vi "Is VI Server Required.vi"(8 "error in (no error)":errorcluster, 11 "Timing Action in":refnum<class "Timing Action.lvclass">) -> (0 "error out":errorcluster, 2 "VI Server Required?":bool, 3 "Timing Action out":refnum<class "Timing Action.lvclass">)   [LabVIEW 2020, in "MacroAssert.lvlib" / "Timing Action.lvclass"]
doc: "Outputs whether VI Server is required to perform the given step."
uses:
  Timing Action.lvclass
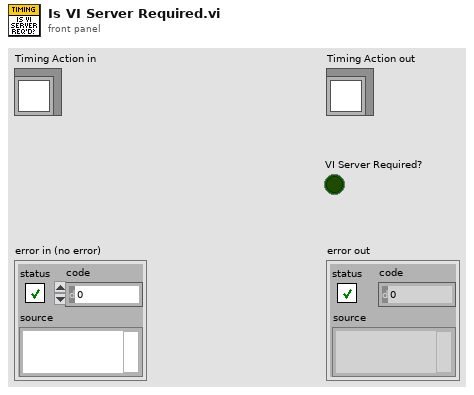
[diagram p1: front panel]
types:
  T1 = typedef "MacroAssert.lvlib/Timing Action.lvclass/Timing Action Type.ctl" = enum16{"Wait", "Wait Until"}
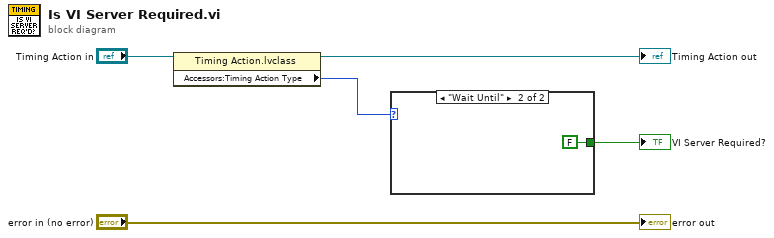
[diagram p0: block diagram]
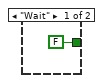
[diagram p2: hidden frame]
diagram:
  n1 = property class="Timing Action.lvclass"(reference="Timing Action in") -> (reference out=→"Timing Action out":refnum<class "Timing Action.lvclass">, "Accessors:Timing Action Type"=w4:T1)  [unwired: 1 in, 1 out]
  n2 = case shown="\"Wait Until\"" w4 {
    tunnel: [FALSE FALSE] -> w1
    frame "Wait" {
    }
    frame "Wait Until" {
    }
  }
  "VI Server Required?" <- w1
  "error out" <- "error in (no error)"
